vi "Integer Wavelet Transform on Image.vi"() -> ()   [LabVIEW 2023]
doc: "This example shows how to perform the integer image decomposition and reconstruction by using the WA Integer Wavelet Transform VI and the WA Inverse Integer Wavelet Transform VI respectively.\n\n<b>Instructions:</b>\n1) Run this VI.\n2) Change the <b>Wavelet</b>, <b>Levels</b>, and <b>Extension</b> settings.\n3) Observe the <b>IWT Coefficients</b> and <b>Reconstructed Image</b>. The <b>Total Difference</b> is zero, because this example can reconstruct the image exactly by using the integer wavelet transform and inverse integer wavelet transform."
uses:
  <vilib>/addons/Wavelet Analysis/typedefs.llb/WA Data.ctl
  <vilib>/addons/Wavelet Analysis/discrete wavelet transform.llb/WA 2D Integer Wavelet Transform.vi
  <vilib>/addons/Wavelet Analysis/discrete wavelet transform.llb/WA Inverse 2D Integer Wavelet Transform.vi
  <vilib>/addons/_Advanced Signal Processing/NI_AdvSigProcWA.lvlib
panel:
  out "Total difference":i32
  in  "Wavelet":u16(ring)=13 items=["Haar"=13, "bior2_2"=16, "bior4_4 (FBI)"=25]
  out "Reconstructed Image":i32[][](graph)
  out "Image":u8[][](graph)
  in  "Extension":u16(ring)=2 items=["Zero padding", "Symmetric", "Periodic"]
  in  "Levels":i32=8
  out "IWT Coefficients":i32[][](graph)
  # "Overview: Shows how to perform the integer image decomposition and reconstruction by using the WA Integer Wavelet Transform VI and the WA Inverse Integer Wavelet Transform VI respectively.\nRequirements: LabVIEW Full Development System, Advanced Signal Processing Toolkit\nInstructions: \n1. Run this VI.\n2. Change the Wavelet, Levels, and Extension settings.\n3. Observe the IWT Coefficients and Reconstructed Image. The Total Difference is zero, because this example can reconstruct the image exactly by using the integer wavelet transform and inverse integer wavelet transform."
  # "IWT"
  # "Encoding"
  # "Inverse IWT"
  # "Decoding"
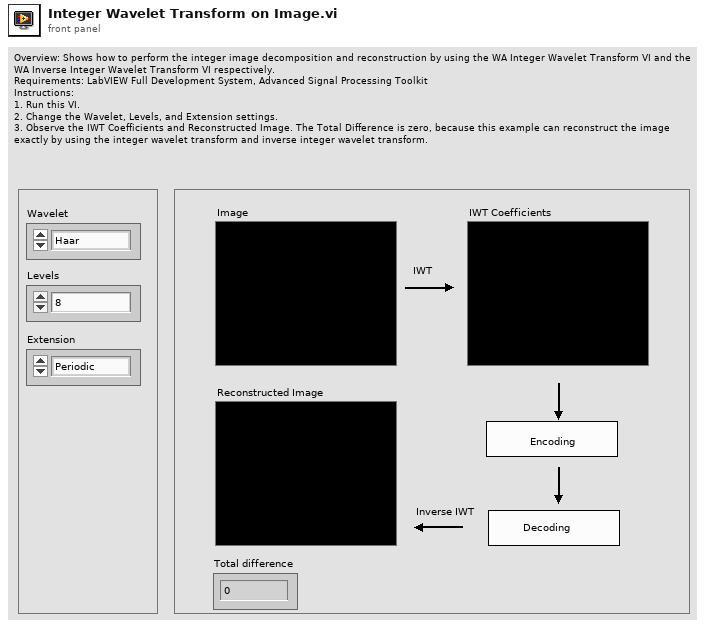
[diagram p1: front panel]
types:
  T1 = typedef "NI_AdvSigProcWA.lvlib/WA Data.ctl" = u16
  T2 = cluster{"low_low":i32[][], "low_high":i32[][], "high_low":i32[][], "high_high":i32[][]}[]
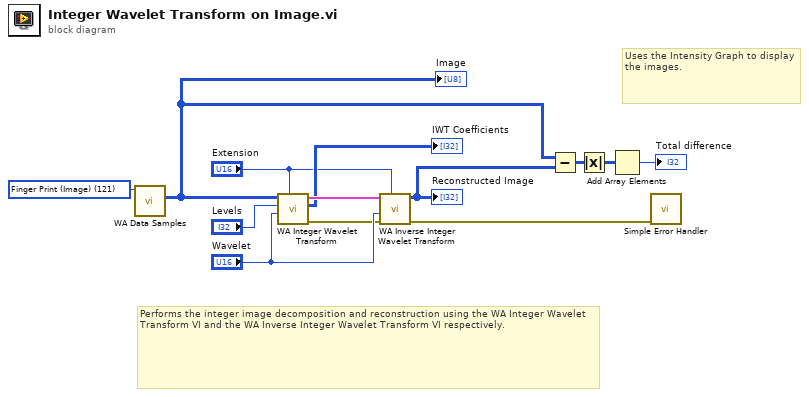
[diagram p0: block diagram]
diagram:
  w3 = T1 121 items=["1D Example Data"=100, "-"=101, "Doppler"=102, "HOP"=103, "TF Sine"=104, "Noisy Doppler"=105, "Sea Temperature"=106, "Sp500"=107, "Power Line"=108, "Engine Knocking"=109, "HeaviSine"=110, "Bumps"=111, "Blocks"=112, "Piece Regular"=113, "HypChirps"=114, "LinChirps"=115, "Chirps"=116, "Piece Polynomial"=117, "ECG"=131, "-"=118, "2D Example Data"=119, "-"=120, "Finger Print (Image)"=121, "Iris Flower (Image)"=122, "Mammogram (Image)"=123, "Lake (Image)"=127, "Two Can 1 (Image)"=132, "Two Can 2 (Image)"=133, "Camera Man (Image)"=134] ("data")
  # "Uses the Intensity Graph to display the images."
  # "Performs the integer image decomposition and reconstruction using the WA Integer Wavelet Transform VI and the WA Inverse Integer Wavelet Transform VI respectively."
  n1 = call <vilib>:"WA Data Samples.vi"("data"=w3) -> ("image"=w8:u8[][])  [unwired: 10 out]
  "Image" <- w8
  n2 = call-poly <vilib>:"WA Integer Wavelet Transform.vi"("extension"="Extension", "wavelet"="Wavelet", "levels"="Levels", "signal"=w8) -> ("error out"=w2:errorcluster, "2D IWT plot"=→"IWT Coefficients":i32[][], "IWT coef"=w13:T2)  [unwired: 1 in, 4 out]
  n3 = call-poly <vilib>:"WA Inverse Integer Wavelet Transform.vi"("extension"="Extension", "error in (no error)"=w2, "wavelet"="Wavelet", "IWT coef"=w13) -> ("error out"=w1:errorcluster, "signal"=w7:i32[][])  [unwired: 6 out]
  "Reconstructed Image" <- w7
  n4 = Subtract(x=w8, y=w7) -> (x-y=w6:i32[][])
  n5 = Absolute Value(x=w6) -> (abs(x)=w5:i32[][])
  n6 = Add Array Elements(numeric array=w5) -> (sum=→"Total difference":i32)
  n7 = call <vilib>:"Simple Error Handler.vi"("error in (no error)"=w1) -> ()  [unwired: 4 in, 5 out]
